vi "相机拍摄图片保存.vi"() -> ()   [LabVIEW 2018]
uses:
  <vilib>/userdefined/High Color/IMAQdx.ctl
  <vilib>/vision/driver/NI_Vision_Acquisition_Software.lvlib
panel:
  in  "保存图片":bool
  out "Image":T1(plugin-control)
  in  "停止":bool
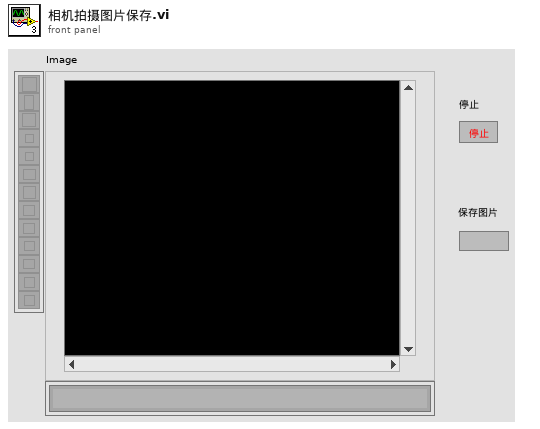
[diagram p1: front panel]
types:
  T1 = typedef "IMAQ Image.ctl" = refnum<image>
  T2 = typedef "IMAQdx.ctl" = refnum<k21>
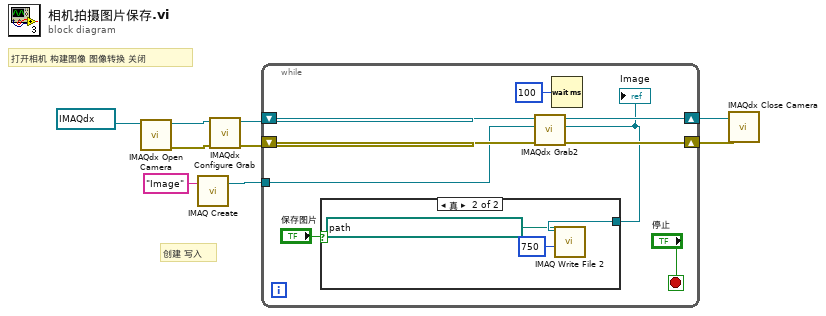
[diagram p0: block diagram]
diagram:
  # "创建 写入"
  # "打开相机 构建图像 图像转换 关闭"
  n1 = call <vilib>:"IMAQdx Open Camera.vi"("Session In"=T2 "cam0") -> ("error out"=w9:errorcluster, "Session Out"=w8:T2)  [unwired: 9 in]
  n2 = call "IMAQ Create"("Image Name"="Image") -> ("New Image"=w3:T1)  [unwired: 4 in, 1 out]
  n3 = call <vilib>:"IMAQdx Configure Grab.vi"("error in"=w9, "Session In"=w8) -> ("error out"=w5:errorcluster, "Session Out"=w7:T2)  [unwired: 8 in]
  n4 = while {
    tunnel: w3 -> [w14]
    shift-right: [w17] -> w6
    shift-left: w7 -> [w18]
    shift-right: [w15] -> w4
    shift-left: w5 -> [w16]
    stop <- "停止" stop-if-true
    n5 = call <vilib>:"IMAQdx Grab2.vi"("error in"=w16, "Image In"=w14, "Session In"=w18) -> ("error out"=w15:errorcluster, "Image Out"=w11:T1, "Session Out"=w17:T2)  [unwired: 5 in, 1 out]
    "Image" <- w11
    n6 = case shown="真" "保存图片" {
      tunnel: w11 -> [_ w21]
      frame False {
      }
      frame True {
        n7 = call-poly "IMAQ Write File 2"("Image Quality"=u32 750, "File Path"=path "D:/Labviewprogram/视觉/1.png", "Image"=w21) -> ()  [unwired: 7 in, 2 out]
      }
    }
    n8 = Wait (ms)(milliseconds to wait=u32 100 ("等待时间（毫秒）")) -> ()  [unwired: 1 out]
  }
  n9 = call <vilib>:"IMAQdx Close Camera.vi"("error in"=w4, "Session In"=w6) -> ()  [unwired: 9 in, 1 out]
